vi "Read FTS Initialization(2).vi"(8 "error in (no error)":errorcluster, 10 "Data Out in":T1={"Message"="", "Homed?"=FALSE, "NextState"=enum."Timeout", "G.Load"=0.0, "G.Position"=0.0, "Load#"=0, "[G.Loads]"=[], "[TotalLoads]"=[], "[Errors]"=[], "ZeroWait"=0, "Results"=[], "DwellWait"=FALSE, "Test Result"=FALSE, "[CondyleLoads]"=[], "[Max]"=[], "[Min]"=[], "Valid String?"=FALSE, "ScanTime"=timestamp(0 s since 1904-01-01), "ScannedString"="", "LabelDevID"=0, "MfgDate"=timestamp(0 s since 1904-01-01), "[EEPROM Cmds]"=[], "[CalData]"=[], "[A/Ds]"=[], "[A/Dmax]"=[], "[A/Dmin]"=[], "BattMax"=0.0, "BattMin"=0.0, "DwellTime"=0, "PendingDeviceType"="", "Zero G.load"=0.0, "GAINC Value"="", "Programming Step"=enum."Load EEPROM", "Front Panel Program?"=FALSE, "Final Program?"=FALSE, "PCB Score"=100, "AssyScore"=100, "Pass/Fail #"="", "Result String"="", "Programming Mode"=enum."Initial Program", "Angle Test Step"=enum."Initialize", "Accel Values"=[], "Shutdown Counter"=0, "V1"=0, "V2"=5, "V3"=0, "V4"=0, "EEPROM Data"=[], "Counter"=0, "Page#"=0, "Timer"=timestamp(0 s since 1904-01-01), "Use Mark10?"=FALSE, "Eng-Result#"=0, "DUT Serial #"=0, "Scroll Message?"=FALSE, "Clear Message"=FALSE, "Batt Test Step "=enum."Initialize", "RXTX Window Found?"=FALSE, "Shutdown First Call?"=FALSE, "A2 Delay (msec)"=500, "Support Script"={"Script #"="", "Script Revision"="", "[OEMs]"=[], "[[DeviceTypes]]"=[], "[[DeviceTypesVals]]"=[], "[[List of Errors]]"=[], "Default GAINC"="", "[[ASICtrims]]"=[], "ID For Echo"="", "Condyle A CalFactor"=100, "Condyle B CalFactor"=100, "[OEMs Prefix]"=[], "Packet ID 18"="", "[[Force Table Load Test]]"=[], "[[Force Table AccurTest]]"=[]}, "Serial Table"={"Serial File Path"=path "", "[[Serial Lookup Table]]"=[], "Serial Device Info"=[], "Valid Serial?"=FALSE}, "Target Information"={"Target Brand"="", "Target DeviceType"="", "Target Serial#"=100, "Target Lot#"=0, "Target DevID"=0, "Target Channel"=5}, "Operator"="", "COM Port"="", "Config Path"=path "", "Tx Array"=[], "DUT Parameters"={"Channel"=0, "DeviceID"=0, "Script Rev"=0, "Month"=0, "Day"=0, "Year"=0, "Lot#"=0, "V1"=0, "V2"=0, "V3"=0, "V4"=0, "MFG"=0, "Cal FactorA"=0, "Cal FactorB"=0, "ASICtrim"=[], "TmpChan"=0, "GAINC"="", "Brand"="", "Device"="", "Serial #"=0, "Batt310"=0, "Batt 280"=0}, "FTS Main?"=FALSE, "Loading"={"[Forces]"=[], "[Dwell]"=[], "Loading Step"=enum."Initialize Test"}, "Software Version"="", "Correction Factor"="", "Second Load Test"=FALSE, "Acc Loads"=[], "Mark10 Config"={"H2S%"=[80.0, 85.0, 90.0, 95.0, 100.0], "H2S Speed"=[12.0, 8.0, 6.0, 4.0, 2.0], "H to S"=2.0, "Home Speed"=1.0, "LoadWin"=0.0, "Load Speed"=0.0, "PID"={"Kp"=0.04, "Kd"=0.005001, "Ki"=2.9999999999999923e-05}}, "Channels"={"Transceiver Ch"=5, "Operating Ch"=5, "Start Ch"=0}} {"Mark10 Config"."PID"."Ki" min=0.0 max=200.0 format="%.6f"; "Mark10 Config"."PID"."Kd" min=0.0 max=200.0 format="%.6f"; "Mark10 Config"."PID"."Kp" min=0.0 max=200.0 format="%.6f"; "DUT Parameters"."ASICtrim" format="%02x"}, 11 "NI_report in":refnum<class "NI_report.lvclass">) -> (0 "error out":errorcluster, 2 "Data Out out":T1={"Message"="", "Homed?"=FALSE, "NextState"=enum."Timeout", "G.Load"=0.0, "G.Position"=0.0, "Load#"=0, "[G.Loads]"=[], "[TotalLoads]"=[], "[Errors]"=[], "ZeroWait"=0, "Results"=[], "DwellWait"=FALSE, "Test Result"=FALSE, "[CondyleLoads]"=[], "[Max]"=[], "[Min]"=[], "Valid String?"=FALSE, "ScanTime"=timestamp(0 s since 1904-01-01), "ScannedString"="", "LabelDevID"=0, "MfgDate"=timestamp(0 s since 1904-01-01), "[EEPROM Cmds]"=[], "[CalData]"=[], "[A/Ds]"=[], "[A/Dmax]"=[], "[A/Dmin]"=[], "BattMax"=0.0, "BattMin"=0.0, "DwellTime"=0, "PendingDeviceType"="", "Zero G.load"=0.0, "GAINC Value"="", "Programming Step"=enum."Load EEPROM", "Front Panel Program?"=FALSE, "Final Program?"=FALSE, "PCB Score"=100, "AssyScore"=100, "Pass/Fail #"="", "Result String"="", "Programming Mode"=enum."Initial Program", "Angle Test Step"=enum."Initialize", "Accel Values"=[], "Shutdown Counter"=0, "V1"=0, "V2"=5, "V3"=0, "V4"=0, "EEPROM Data"=[], "Counter"=0, "Page#"=0, "Timer"=timestamp(0 s since 1904-01-01), "Use Mark10?"=FALSE, "Eng-Result#"=0, "DUT Serial #"=0, "Scroll Message?"=FALSE, "Clear Message"=FALSE, "Batt Test Step "=enum."Initialize", "RXTX Window Found?"=FALSE, "Shutdown First Call?"=FALSE, "A2 Delay (msec)"=500, "Support Script"={"Script #"="", "Script Revision"="", "[OEMs]"=[], "[[DeviceTypes]]"=[], "[[DeviceTypesVals]]"=[], "[[List of Errors]]"=[], "Default GAINC"="", "[[ASICtrims]]"=[], "ID For Echo"="", "Condyle A CalFactor"=100, "Condyle B CalFactor"=100, "[OEMs Prefix]"=[], "Packet ID 18"="", "[[Force Table Load Test]]"=[], "[[Force Table AccurTest]]"=[]}, "Serial Table"={"Serial File Path"=path "", "[[Serial Lookup Table]]"=[], "Serial Device Info"=[], "Valid Serial?"=FALSE}, "Target Information"={"Target Brand"="", "Target DeviceType"="", "Target Serial#"=100, "Target Lot#"=0, "Target DevID"=0, "Target Channel"=5}, "Operator"="", "COM Port"="", "Config Path"=path "", "Tx Array"=[], "DUT Parameters"={"Channel"=0, "DeviceID"=0, "Script Rev"=0, "Month"=0, "Day"=0, "Year"=0, "Lot#"=0, "V1"=0, "V2"=0, "V3"=0, "V4"=0, "MFG"=0, "Cal FactorA"=0, "Cal FactorB"=0, "ASICtrim"=[], "TmpChan"=0, "GAINC"="", "Brand"="", "Device"="", "Serial #"=0, "Batt310"=0, "Batt 280"=0}, "FTS Main?"=FALSE, "Loading"={"[Forces]"=[], "[Dwell]"=[], "Loading Step"=enum."Initialize Test"}, "Software Version"="", "Correction Factor"="", "Second Load Test"=FALSE, "Acc Loads"=[], "Mark10 Config"={"H2S%"=[80.0, 85.0, 90.0, 95.0, 100.0], "H2S Speed"=[12.0, 8.0, 6.0, 4.0, 2.0], "H to S"=2.0, "Home Speed"=1.0, "LoadWin"=0.0, "Load Speed"=0.0, "PID"={"Kp"=0.04, "Kd"=0.005001, "Ki"=2.9999999999999923e-05}}, "Channels"={"Transceiver Ch"=5, "Operating Ch"=5, "Start Ch"=0}} {"Mark10 Config"."PID"."Ki" min=0.0 max=200.0 format="%.6f"; "Mark10 Config"."PID"."Kd" min=0.0 max=200.0 format="%.6f"; "Mark10 Config"."PID"."Kp" min=0.0 max=200.0 format="%.6f"; "DUT Parameters"."ASICtrim" format="%02x"}, 3 "report out":refnum<class "NI_report.lvclass">)   [LabVIEW 2013]
uses:
  <vilib>/addons/_office/NI_ReportGenerationToolkit.lvlib
  <vilib>/addons/_office/excel.llb/Excel Get Data ([str]).vi
  <vilib>/Utility/NIReport.llb/Excel/NI_Excel.lvclass
  <vilib>/addons/_office/excel.llb/Excel Get Data ([dbl]).vi
  <vilib>/addons/_office/excel.llb/Excel Get Data (str).vi
  <vilib>/addons/_office/excel.llb/Excel Get Data (i32).vi
  <vilib>/addons/_office/excel.llb/Excel Get Data (dbl).vi
  Controls/Load Step.ctl
  Controls/Gen2 FT states.ctl
  Controls/Iniial Device Programming.ctl
  SubVI/ProgramStageControl.ctl
  Controls/Batt Cap Steps.ctl
  Controls/Support Script.ctl
  Controls/Serial Table.ctl
  Controls/Device Information.ctl
  Controls/InfoPacket.ctl
  Controls/LocalVars.ctl
  <vilib>/Utility/NIReport.llb/NI_report.lvclass
  Controls/Loading.ctl
  Controls/PID parameters.ctl
  Controls/Mark10 Config.ctl
  Controls/Channels.ctl
panel:
  out "Acc Test":dbl[][](array[numeric]) format="%.2f"
  out "Load Test":dbl[][](array[numeric]) format="%.2f"
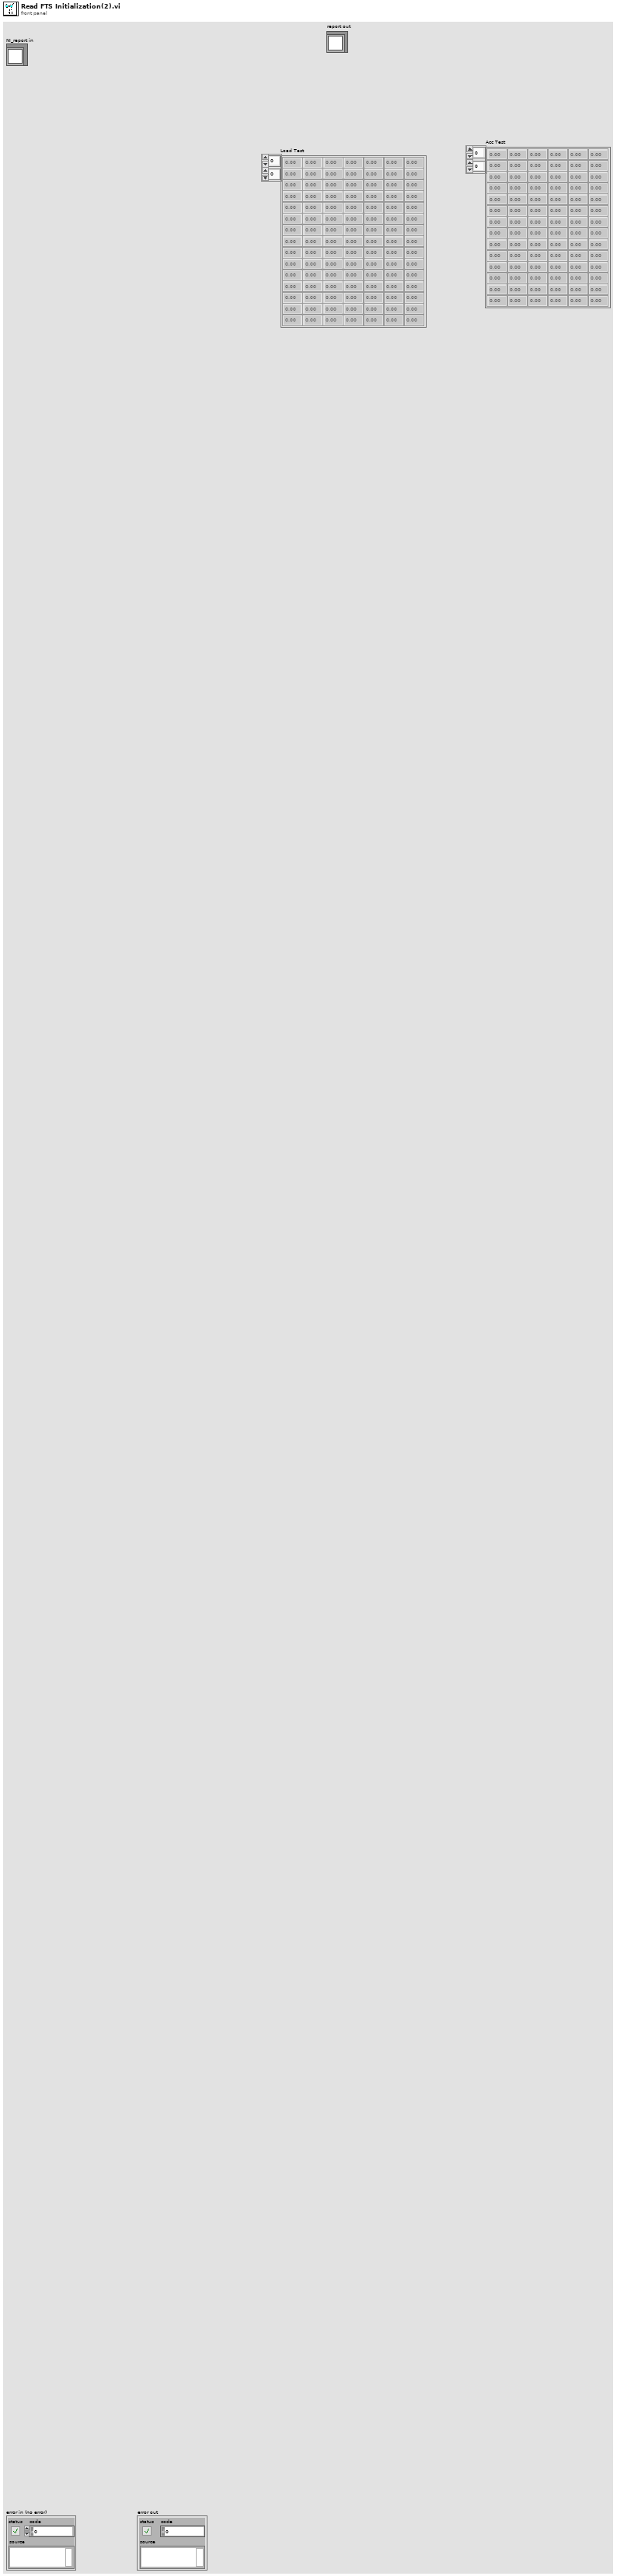
[diagram p1: front panel]
types:
  T1 = typedef "LocalVars.ctl" = cluster{"Message":string, "Homed?":bool, "NextState":T2, "G.Load":dbl, "G.Position":dbl, "Load#":i32, "[G.Loads]":dbl[], "[TotalLoads]":dbl[], "[Errors]":dbl[][], "ZeroWait":u32, "Results":dbl[], "DwellWait":bool, "Test Result":bool, "[CondyleLoads]":dbl[][], "[Max]":dbl[], "[Min]":dbl[], "Valid String?":bool, "ScanTime":timestamp, "ScannedString":string, "LabelDevID":u32, "MfgDate":timestamp, "[EEPROM Cmds]":u8[][], "[CalData]":u8[][], "[A/Ds]":dbl[][], "[A/Dmax]":dbl[], "[A/Dmin]":dbl[], "BattMax":dbl, "BattMin":dbl, "DwellTime":i32, "PendingDeviceType":string, "Zero G.load":dbl, "GAINC Value":string, "Programming Step":T3, "Front Panel Program?":bool, "Final Program?":bool, "PCB Score":i32, "AssyScore":i32, "Pass/Fail #":string, "Result String":string, "Programming Mode":T4, "Angle Test Step":enum16{"Initialize", "Get X", "Get Y", "Get Z", "Next Test"}, "Accel Values":dbl[][], "Shutdown Counter":u32, "V1":i32, "V2":i32, "V3":i32, "V4":i32, "EEPROM Data":i32[][], "Counter":i32, "Page#":i32, "Timer":timestamp, "Use Mark10?":bool, "Eng-Result#":u32, "DUT Serial #":i32, "Scroll Message?":bool, "Clear Message":bool, "Batt Test Step ":T5, "RXTX Window Found?":bool, "Shutdown First Call?":bool, "A2 Delay (msec)":i16, "Support Script":T6, "Serial Table":T7, "Target Information":T8, "Operator":string, "COM Port":string, "Config Path":path, "Tx Array":u8[], "DUT Parameters":T9, "FTS Main?":bool, "Loading":T10, "Software Version":string, "Correction Factor":string, "Second Load Test":bool, "Acc Loads":dbl[][], "Mark10 Config":T12, "Channels":T14}
  T2 = typedef "Gen2 FT states.ctl" = enum16{"---------SETUP-------", "Initialization", "Read Support Data", "Initialize Mark-10", "Initialize Transceiver", "------UTILITIES------", "Change DUT Channel", "Find RxTx Window", "Reset Device", "Scan Channels", "Read Serial Lookup", "Shutdown Device", "ESTOP", "--------USER---------", "Timeout", "-----PROGRAM-----", "Program Device", "------MARK10--------", "Go Home", "MoveUp", "MoveDown", "Goto Load", "Goto Position", "Stop Motor", "---------TESTS--------", "Start Test", "Angle Test", "Load Test", "Load Accuracy Test", "Battery Test", "------RESULTS-------", "End Test", "Display Result", "--------EXIT--------", "Exit"}
  T3 = typedef "Iniial Device Programming.ctl" = enum16{"Load EEPROM", "Send First A1", "Send EEPROM", "Send A1", "Check EEPROM Echo", "Verify transmission", "Programming Successful", "Programming Failed"}
  T4 = typedef "ProgramStageControl.ctl" = enum16{"Initial Program", "GainC", "Scales"}
  T5 = typedef "Batt Cap Steps.ctl" = enum16{"Initialize", "Collect 2.8 Volts", "Collect 3.1 Volts", "Check Results"}
  T6 = typedef "Support Script.ctl" = cluster{"Script #":string, "Script Revision":string, "[OEMs]":string[], "[[DeviceTypes]]":string[][], "[[DeviceTypesVals]]":u16[][], "[[List of Errors]]":string[][], "Default GAINC":string, "[[ASICtrims]]":u8[][], "ID For Echo":string, "Condyle A CalFactor":i32, "Condyle B CalFactor":i32, "[OEMs Prefix]":string[], "Packet ID 18":string, "[[Force Table Load Test]]":dbl[][], "[[Force Table AccurTest]]":dbl[][]}
  T7 = typedef "Serial Table.ctl" = cluster{"Serial File Path":path, "[[Serial Lookup Table]]":string[][], "Serial Device Info":string[], "Valid Serial?":bool}
  T8 = typedef "Device Information.ctl" = cluster{"Target Brand":string, "Target DeviceType":string, "Target Serial#":i32, "Target Lot#":u32, "Target DevID":u32, "Target Channel":u8}
  T9 = typedef "InfoPacket.ctl" = cluster{"Channel":u8, "DeviceID":u32, "Script Rev":u8, "Month":u8, "Day":u8, "Year":u8, "Lot#":u32, "V1":u16, "V2":u16, "V3":u16, "V4":u16, "MFG":u8, "Cal FactorA":u8, "Cal FactorB":u8, "ASICtrim":u8[], "TmpChan":u8, "GAINC":string, "Brand":string, "Device":string, "Serial #":u64, "Batt310":u16, "Batt 280":u16}
  T10 = typedef "Loading.ctl" = cluster{"[Forces]":dbl[], "[Dwell]":dbl[], "Loading Step":T11}
  T11 = typedef "Load Step.ctl" = enum16{"Initialize Test", "Go Home", "Detect Dev Surface", "Wait to zero Device", "Zero Device", "Do Test", "Test Result"}
  T12 = typedef "Mark10 Config.ctl" = cluster{"H2S%":dbl[], "H2S Speed":dbl[], "H to S":dbl, "Home Speed":dbl, "LoadWin":dbl, "Load Speed":dbl, "PID":T13}
  T13 = typedef "PID parameters.ctl" = cluster{"Kp":dbl, "Kd":dbl, "Ki":dbl}
  T14 = typedef "Channels.ctl" = cluster{"Transceiver Ch":u8, "Operating Ch":u8, "Start Ch":u8}
  T15 = cluster{"data[0]":dbl, "data[1]":dbl, "data[2]":dbl, "data[3]":dbl, "data[4]":dbl, "data[5]":dbl, "data[6]":dbl, "data[7]":dbl, "data[8]":dbl}
  T16 = cluster{"data[0]":dbl, "data[1]":dbl, "data[2]":dbl, "data[3]":dbl}
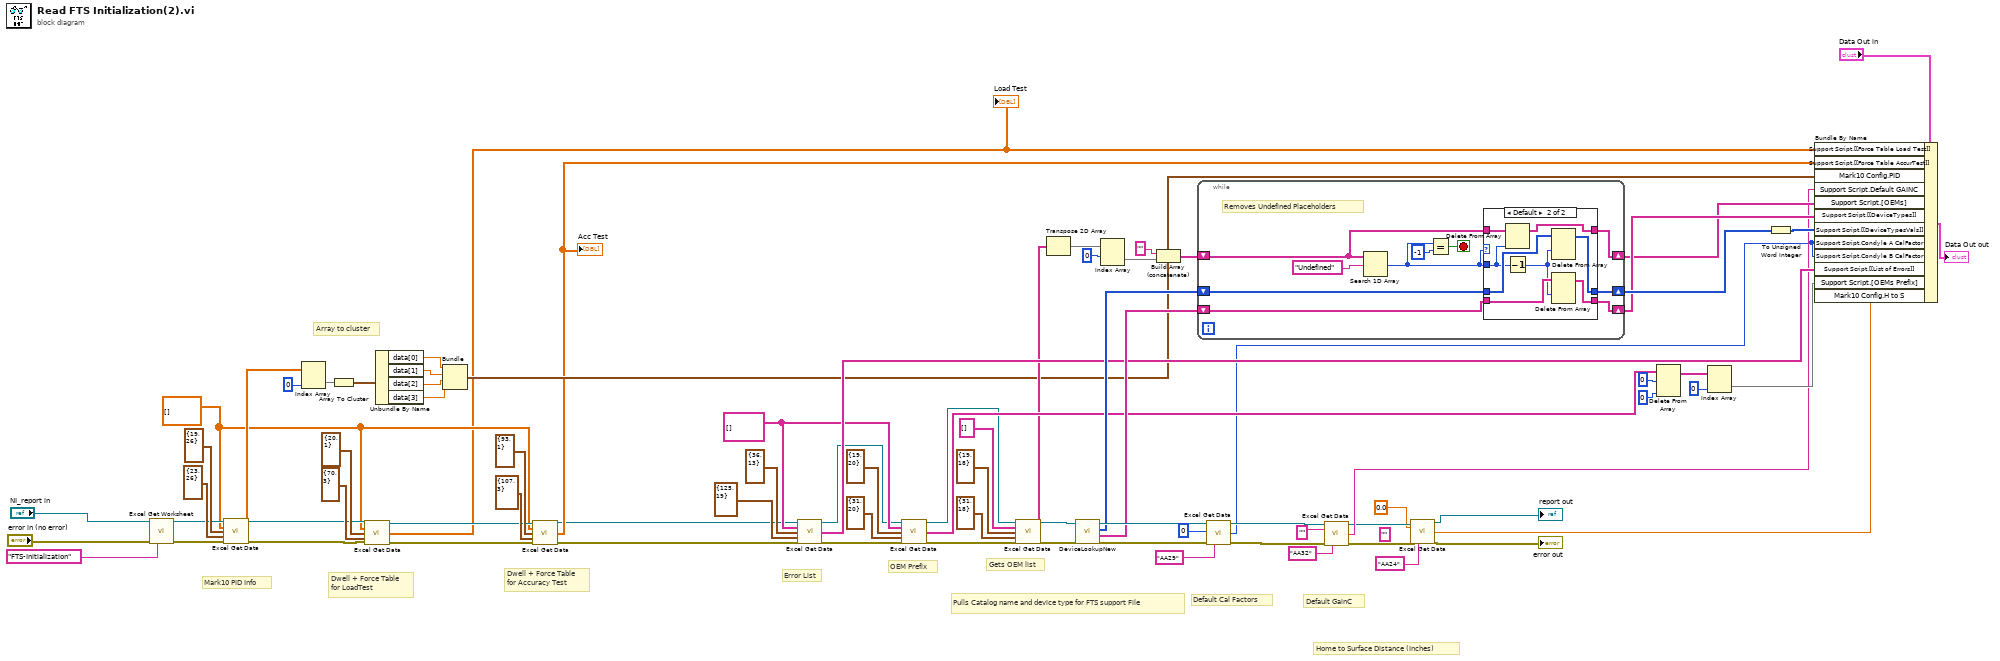
[diagram p0: block diagram]
diagram:
  (unwired) ""
  w12 = dbl[][] [] ("data type")
  w59 = string[][] [] ("data type")
  # "Home to Surface Distance (Inches)"
  # "Dwell + Force Table\nfor Accuracy Test"
  # "Dwell + Force Table\nfor LoadTest"
  # "Mark10 PID Info"
  # "Array to cluster"
  # "Pulls Catalog name and device type for FTS support File"
  # "Default GainC"
  # "Error List"
  # "Default Cal Factors"
  # "OEM Prefix"
  # "Gets OEM list"
  n1 = call <vilib>:"Excel Get Worksheet.vi"("report in"="NI_report in", "error in (no error)"="error in (no error)", "name (\"\")"="FTS-Initialization" ("name (\"\")")) -> ("report out"=w20:refnum<class "NI_report.lvclass">, "error out"=w21:errorcluster)  [unwired: 11 in]
  n2 = call-poly <vilib>:"Excel Get Data.vi"("report in"=w20, "data type"=w12, "start (-1, -1)"=cluster{"row":i32, "column":i32} {"row"=19, "column"=26}, "end (-1, -1)"=cluster{"row":i32, "column":i32} {"row"=23, "column"=26}, "error in (no error)"=w21) -> ("report out"=w16:refnum<class "NI_report.lvclass">, "data"=w25:dbl[][], "error out"=w15:errorcluster)  [unwired: 8 in]
  n3 = Index Array(array=w25, index (col)=0 ("index (row)")) -> (element=w32:dbl[])  [unwired: 1 in]
  n4 = Array To Cluster(array=w32) -> (cluster=w27:T15)
  n5 = call-poly <vilib>:"Excel Get Data.vi"("report in"=w16, "data type"=w12, "start (-1, -1)"=cluster{"row":i32, "column":i32} {"row"=20, "column"=1}, "end (-1, -1)"=cluster{"row":i32, "column":i32} {"row"=70, "column"=3} ("start (-1, -1)"), "error in (no error)"=w15) -> ("report out"=w13:refnum<class "NI_report.lvclass">, "data"=w11:dbl[][], "error out"=w14:errorcluster)  [unwired: 8 in]
  "Load Test" <- w11
  n6 = Unbundle By Name(w27) -> ("data[0]"=w28:dbl, "data[1]"=w29:dbl, "data[2]"=w30:dbl, "data[3]"=w31:dbl)
  n7 = Bundle("data[0]"=w28, "data[1]"=w29, "data[2]"=w30, "data[3]"=w31) -> (w22:T16)  [unwired: 1 in]
  n8 = call-poly <vilib>:"Excel Get Data.vi"("report in"=w13, "data type"=w12, "start (-1, -1)"=cluster{"row":i32, "column":i32} {"row"=93, "column"=1}, "end (-1, -1)"=cluster{"row":i32, "column":i32} {"row"=107, "column"=3} ("start (-1, -1)"), "error in (no error)"=w14) -> ("report out"=w8:refnum<class "NI_report.lvclass">, "data"=w10:dbl[][], "error out"=w9:errorcluster)  [unwired: 8 in]
  "Acc Test" <- w10
  n9 = call-poly <vilib>:"Excel Get Data.vi"("report in"=w8, "data type"=w59, "start (-1, -1)"=cluster{"row":i32, "column":i32} {"row"=36, "column"=13}, "end (-1, -1)"=cluster{"row":i32, "column":i32} {"row"=125, "column"=19}, "error in (no error)"=w9) -> ("report out"=w57:refnum<class "NI_report.lvclass">, "data"=w64:string[][], "error out"=w55:errorcluster)  [unwired: 8 in]
  n10 = call-poly <vilib>:"Excel Get Data.vi"("report in"=w57, "data type"=w59, "start (-1, -1)"=cluster{"row":i32, "column":i32} {"row"=19, "column"=20}, "end (-1, -1)"=cluster{"row":i32, "column":i32} {"row"=31, "column"=20}, "error in (no error)"=w55) -> ("report out"=w58:refnum<class "NI_report.lvclass">, "data"=w70:string[][], "error out"=w56:errorcluster)  [unwired: 8 in]
  n11 = call-poly <vilib>:"Excel Get Data.vi"("report in"=w58, "data type"=string[][] [], "start (-1, -1)"=cluster{"row":i32, "column":i32} {"row"=19, "column"=18}, "end (-1, -1)"=cluster{"row":i32, "column":i32} {"row"=31, "column"=18}, "error in (no error)"=w56) -> ("report out"=w37:refnum<class "NI_report.lvclass">, "data"=w44:string[][], "error out"=w38:errorcluster)  [unwired: 8 in]
  n12 = Transpose 2D Array(2D array=w44) -> (transposed array=w45:string[][])
  n13 = call "DeviceLookupNew.vi"("error in (no error)"=w38, "report in"=w37) -> ("error out"=w80:errorcluster, "[[Device Types]]"=w77:string[][], "[[DeviceTypesVals]]"=w78:i32[][], "report out"=w79:refnum<class "NI_report.lvclass">)  [unwired: 2 in]
  n14 = Index Array(array=w45, index (row)=0) -> (element=w49:string[])  [unwired: 1 in]
  n15 = Build Array (concatenate)("", w49) -> (w51:string[])
  n16 = while {
    shift-right: [w91] -> w63
    shift-left: w51 -> [w88]
    shift-right: [w90] -> w65
    shift-left: w77 -> [w82]
    shift-right: [w83] -> w66
    shift-left: w78 -> [w84]
    stop <- w87 stop-if-true
    # "Removes Undefined Placeholders"
    n17 = Search 1D Array(1D array=w88, element="Undefined") -> (index of element=w85:i32)  [unwired: 1 in]
    n18 = Equal?(x=w85, y=-1) -> (x = y?=w87:bool)
    n19 = case shown="Default" w85 {
      tunnel: w82 -> [w93 w99]
      tunnel: [w94 w102] -> w91
      tunnel: [w93 w101] -> w90
      tunnel: w85 -> [_ w96]
      tunnel: w88 -> [w94 w100]
      tunnel: w84 -> [w92 w98]
      tunnel: [w92 w97] -> w83
      frame -1 {
      }
      frame Default {
        n20 = Delete From Array(array=w100, index=w96) -> (array with subset deleted=w102:string[])  [unwired: 1 in, 1 out]
        n21 = Decrement(x=w96) -> (x-1=w95:i32)
        n22 = Delete From Array(array=w98, index (row)=w95) -> (array with subset deleted=w97:i32[][])  [unwired: 2 in, 1 out]
        n23 = Delete From Array(array=w99, index (row)=w95) -> (array with subset deleted=w101:string[][])  [unwired: 2 in, 1 out]
      }
    }
  }
  n24 = call-poly <vilib>:"Excel Get Data.vi"("report in"=w79, "data type"=0, "error in (no error)"=w80, "name (\"\")"="AA29" ("name (\"\")")) -> ("report out"=w46:refnum<class "NI_report.lvclass">, "data"=w17:i32, "error out"=w47:errorcluster)  [unwired: 9 in]
  n25 = call-poly <vilib>:"Excel Get Data.vi"("report in"=w46, "data type"="", "error in (no error)"=w47, "name (\"\")"="AA32" ("name (\"\")")) -> ("report out"=w7:refnum<class "NI_report.lvclass">, "data"=w62:string, "error out"=w5:errorcluster)  [unwired: 9 in]
  n26 = call-poly <vilib>:"Excel Get Data.vi"("report in"=w7, "data type"=0.0, "error in (no error)"=w5, "name (\"\")"="AA24" ("name (\"\")")) -> ("report out"=→"report out":refnum<class "NI_report.lvclass">, "data"=w1:dbl, "error out"=→"error out":errorcluster)  [unwired: 9 in]
  n27 = Delete From Array(array=w70, length=0, index (col)=0 ("index (row)")) -> (array with subset deleted=w72:string[][])  [unwired: 1 in, 1 out]
  n28 = Index Array(array=w72, index (col)=0 ("disabled index (col)")) -> (element=w68:string[])  [unwired: 1 in]
  n29 = To Unsigned Word Integer(number=w66) -> (unsigned 16bit integer=w67:u16[][])
  n30 = Bundle By Name(cluster="Data Out in", "Support Script.[[Force Table Load Test]]"=w11, "Support Script.[[Force Table AccurTest]]"=w10, "Mark10 Config.PID"=w22, "Support Script.Default GAINC"=w62, "Support Script.[OEMs]"=w63, "Support Script.[[DeviceTypes]]"=w65, "Support Script.[[DeviceTypesVals]]"=w67, "Support Script.Condyle A CalFactor"=w17, "Support Script.Condyle B CalFactor"=w17, "Support Script.[[List of Errors]]"=w64, "Support Script.[OEMs Prefix]"=w68, "Mark10 Config.H to S"=w1) -> (→"Data Out out":T1)
